vi "test.vi"   [LabVIEW 2019]
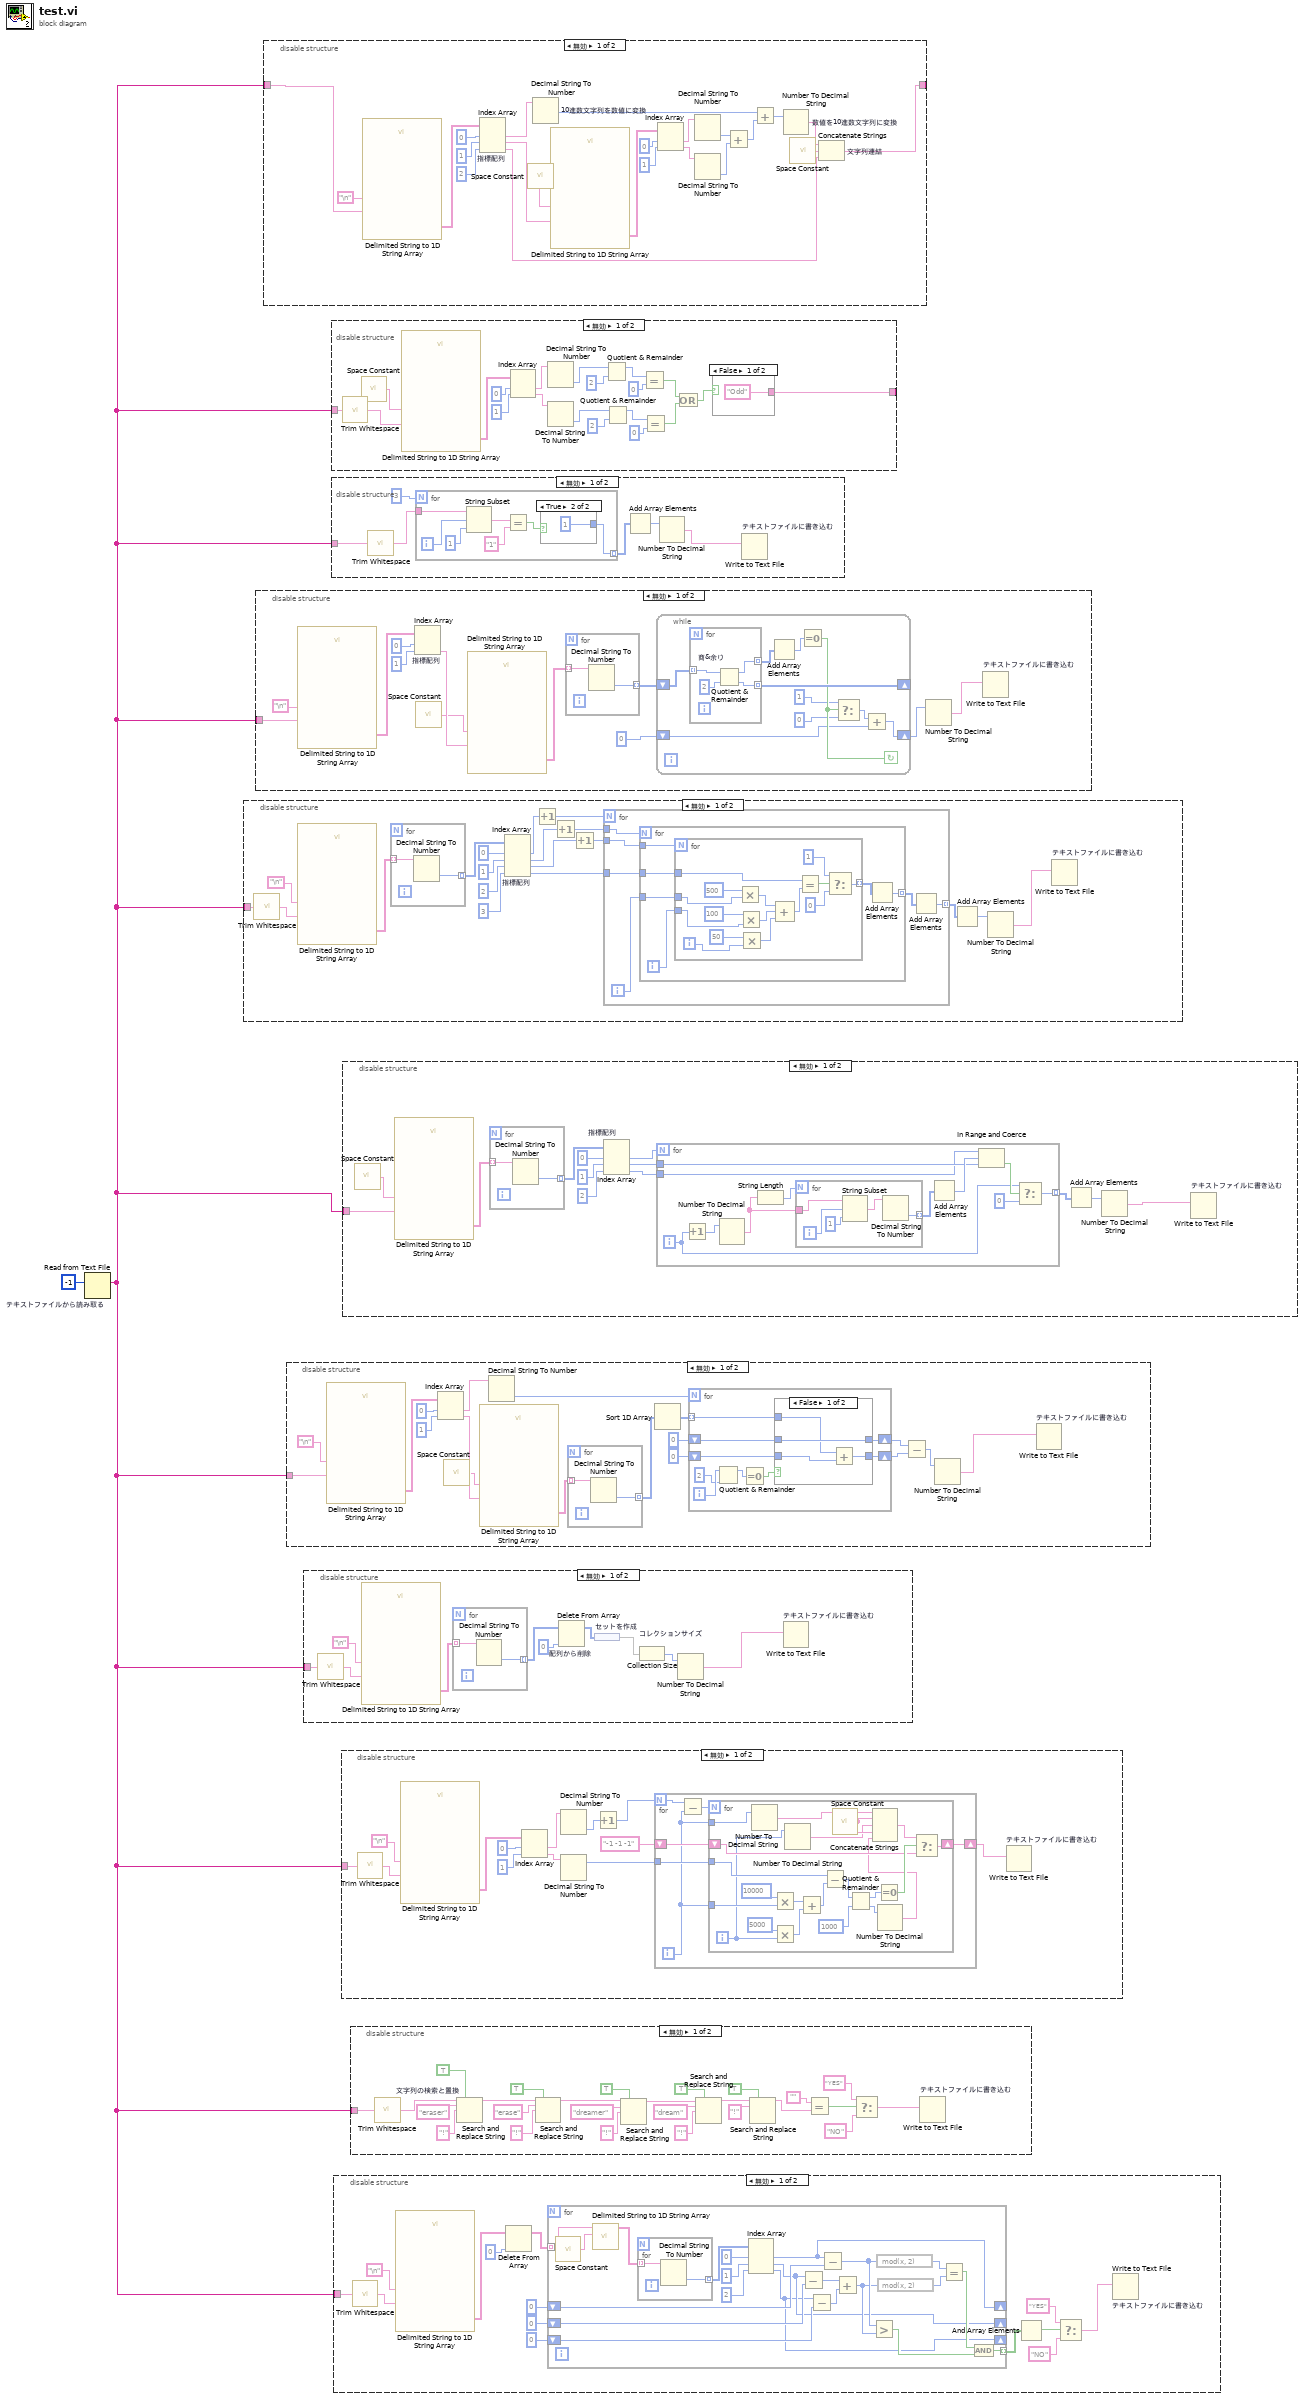
[diagram p0: block diagram]
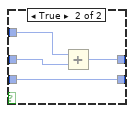
[diagram p7: hidden frame]
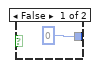
[diagram p11: hidden frame]
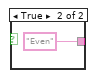
[diagram p13: hidden frame]
diagram:
  n1 = Read from Text File "テキストファイルから読み取る"(count=-1) -> (text=w1:string)  [unwired: 3 in, 3 out]
  n2 = disable-structure shown="無効" {
    disable-tunnel: w1 -> [w21 _]
    frame Disabled {
      n3 = call <vilib>:"Trim Whitespace.vi"("string"=w21) -> ("trimmed string"=w16:string)  [unwired: 1 in]
      n4 = call <vilib>:"Delimited String to 1D String Array.vi"("delimiter"="\n", "delimited string"=w16) -> ("string array"=w13:string[])  [unwired: 9 in]
      n5 = for {
        tunnel: w13 -> [w50] mode=indexing
        tunnel: [w49] -> w12 mode=indexing
        n6 = Decimal String To Number(string=w50) -> (number=w49:i32)  [unwired: 2 in, 1 out]
      }
      n7 = Index Array "指標配列"(array=w12, index #1=0, index #2=1, index #3=2, index #4=3) -> (element #1=w8:i32, element #2=w6:i32, element #3=w4:i32, element #4=w11:i32)
      n8 = Increment(x=w8) -> (x+1=w7:i32)
      n9 = Increment(x=w6) -> (x+1=w5:i32)
      n10 = Increment(x=w4) -> (x+1=w3:i32)
      n11 = for {
        N: w7 -> [_]
        tunnel: w5 -> [w27]
        tunnel: w3 -> [w26]
        tunnel: w11 -> [w25]
        tunnel: [w22] -> w10 mode=indexing
        i -> [w24]
        n12 = for {
          N: w27 -> [_]
          tunnel: w26 -> [w33]
          tunnel: w25 -> [w32]
          tunnel: w24 -> [w31]
          tunnel: [w28] -> w23 mode=indexing
          i -> [w30]
          n13 = for {
            N: w33 -> [_]
            tunnel: w32 -> [w39]
            tunnel: w31 -> [w47]
            tunnel: w30 -> [w45]
            tunnel: [w35] -> w29 mode=indexing
            i -> [w43]
            n14 = Multiply(x=500, y=w47) -> (x*y=w42:i32)
            n15 = Multiply(x=100, y=w45) -> (x*y=w41:i32)
            n16 = Multiply(x=50, y=w43) -> (x*y=w40:i32)
            n17 = Compound Arithmetic op=ADD(w42, w41, w40) -> (w34:i32)
            n18 = Equal?(x=w39, y=w34) -> (x = y?=w38:bool)
            n19 = Select(t=1, s=w38, f=0) -> (s? t:f=w35:i32)
          }
          n20 = Add Array Elements(numeric array=w29) -> (sum=w28:i32)
        }
        n21 = Add Array Elements(numeric array=w23) -> (sum=w22:i32)
      }
      n22 = Add Array Elements(numeric array=w10) -> (sum=w9:i32)
      n23 = Number To Decimal String(number=w9) -> (decimal integer string=w20:string)  [unwired: 1 in]
      n24 = Write to Text File "テキストファイルに書き込む"(text=w20) -> ()  [unwired: 3 in, 3 out]
    }
    frame Enabled {
    }
  }
  n25 = disable-structure shown="無効" {
    disable-tunnel: w1 -> [w62 _]
    frame Disabled {
      n26 = call <vilib>:"Delimited String to 1D String Array.vi"("delimiter"="\n", "delimited string"=w62) -> ("string array"=w57:string[])  [unwired: 9 in]
      n27 = Index Array "指標配列"(array=w57, index #1=0, index #2=1) -> (element #2=w56:string)  [unwired: 1 out]
      n28 = call <vilib>:"Space Constant.vi"() -> ("String"=w55:string)
      n29 = call <vilib>:"Delimited String to 1D String Array.vi"("delimiter"=w55, "delimited string"=w56) -> ("string array"=w54:string[])  [unwired: 9 in]
      n30 = for {
        tunnel: w54 -> [w64] mode=indexing
        tunnel: [w63] -> w53 mode=indexing
        n31 = Decimal String To Number(string=w64) -> (number=w63:i32)  [unwired: 2 in, 1 out]
      }
      n32 = while {
        shift-right: [w72] -> _
        shift-left: w53 -> [w74]
        shift-right: [w65] -> w51
        shift-left: 0 -> [w66]
        stop <- w70 continue-if-true
        n33 = for {
          tunnel: w74 -> [w78] mode=indexing
          tunnel: [w76] -> w72 mode=indexing
          tunnel: [w75] -> w73 mode=indexing
          n34 = Quotient & Remainder "商&余り"(x=w78, y=2) -> (x-y*floor(x/y)=w75:i32, floor(x/y)=w76:i32)
        }
        n35 = Add Array Elements(numeric array=w73) -> (sum=w71:i32)
        n36 = Equal To 0?(x=w71) -> (x = 0?=w70:bool)
        n37 = Select(t=1, s=w70, f=0) -> (s? t:f=w67:i32)
        n38 = Add(x=w67, y=w66) -> (x+y=w65:i32)
      }
      n39 = Number To Decimal String(number=w51) -> (decimal integer string=w61:string)  [unwired: 1 in]
      n40 = Write to Text File "テキストファイルに書き込む"(text=w61) -> ()  [unwired: 3 in, 3 out]
    }
    frame Enabled {
    }
  }
  n41 = disable-structure shown="無効" {
    disable-tunnel: w1 -> [w101 _]
    disable-tunnel: [w79 _] -> _
    frame Disabled {
      n42 = call <vilib>:"Delimited String to 1D String Array.vi"("delimiter"="\n", "delimited string"=w101) -> ("string array"=w100:string[])  [unwired: 9 in]
      n43 = Index Array "指標配列"(array=w100, index #1=0, index #2=1, index #3=2) -> (element #1=w95:string, element #2=w94:string, element #3=w80:string)
      n44 = call <vilib>:"Space Constant.vi"() -> ("String"=w93:string)
      n45 = Decimal String To Number "10進数文字列を数値に変換"(string=w95) -> (number=w86:i32)  [unwired: 2 in, 1 out]
      n46 = call <vilib>:"Delimited String to 1D String Array.vi"("delimiter"=w93, "delimited string"=w94) -> ("string array"=w92:string[])  [unwired: 9 in]
      n47 = Index Array(array=w92, index #1=0, index #2=1) -> (element #1=w89:string, element #2=w88:string)
      n48 = Decimal String To Number(string=w89) -> (number=w85:i32)  [unwired: 2 in, 1 out]
      n49 = Decimal String To Number(string=w88) -> (number=w84:i32)  [unwired: 2 in, 1 out]
      n50 = Add(x=w85, y=w84) -> (x+y=w87:i32)
      n51 = Add(x=w86, y=w87) -> (x+y=w83:i32)
      n52 = Number To Decimal String "数値を10進数文字列に変換"(number=w83) -> (decimal integer string=w82:string)  [unwired: 1 in]
      n53 = call <vilib>:"Space Constant.vi"() -> ("String"=w81:string)
      n54 = Concatenate Strings "文字列連結"(w82, w81, w80) -> (w79:string)
    }
    frame Enabled {
    }
  }
  n55 = disable-structure shown="無効" {
    disable-tunnel: w1 -> [w118 _]
    frame Disabled {
      n56 = call <vilib>:"Delimited String to 1D String Array.vi"("delimiter"="\n", "delimited string"=w118) -> ("string array"=w117:string[])  [unwired: 9 in]
      n57 = Index Array ("指標配列")(array=w117, index #1=0, index #2=1) -> (element #1=w113:string, element #2=w112:string)
      n58 = call <vilib>:"Space Constant.vi"() -> ("String"=w111:string)
      n59 = call <vilib>:"Delimited String to 1D String Array.vi"("delimiter"=w111, "delimited string"=w112) -> ("string array"=w110:string[])  [unwired: 9 in]
      n60 = Decimal String To Number(string=w113) -> (number=w109:i32)  [unwired: 2 in, 1 out]
      n61 = for {
        tunnel: w110 -> [w121] mode=indexing
        tunnel: [w120] -> w108 mode=indexing
        n62 = Decimal String To Number(string=w121) -> (number=w120:i32)  [unwired: 2 in, 1 out]
      }
      n63 = Sort 1D Array(array=w108) -> (sorted array=w107:i32[])
      n64 = for {
        N: w109 -> [_]
        tunnel: w107 -> [w123] mode=indexing
        shift-right: [w126] -> w104
        shift-left: 0 -> [w127]
        shift-right: [w124] -> w103
        shift-left: 0 -> [w125]
        i -> [w130]
        n65 = Quotient & Remainder(x=w130, y=2) -> (x-y*floor(x/y)=w129:i32)  [unwired: 1 out]
        n66 = Equal To 0?(x=w129) -> (x = 0?=w128:bool)
        n67 = case shown="FALSE" w128 {
          tunnel: w127 -> [w134 w138]
          tunnel: [w134 w136] -> w126
          tunnel: w125 -> [w133 w137]
          tunnel: [w132 w137] -> w124
          tunnel: w123 -> [w131 w135]
          frame False {
            n68 = Add(x=w131, y=w133) -> (x+y=w132:i32)
          }
          frame True {
            n69 = Add(x=w135, y=w138) -> (x+y=w136:i32)
          }
        }
      }
      n70 = Subtract(x=w104, y=w103) -> (x-y=w102:i32)
      n71 = Number To Decimal String(number=w102) -> (decimal integer string=w119:string)  [unwired: 1 in]
      n72 = Write to Text File "テキストファイルに書き込む"(text=w119) -> ()  [unwired: 3 in, 3 out]
    }
    frame Enabled {
    }
  }
  n73 = disable-structure shown="無効" {
    disable-tunnel: w1 -> [w147 _]
    frame Disabled {
      n74 = call <vilib>:"Trim Whitespace.vi"("string"=w147) -> ("trimmed string"=w146:string)  [unwired: 1 in]
      n75 = call <vilib>:"Delimited String to 1D String Array.vi"("delimiter"="\n", "delimited string"=w146) -> ("string array"=w143:string[])  [unwired: 9 in]
      n76 = for {
        tunnel: w143 -> [w150] mode=indexing
        tunnel: [w149] -> w142 mode=indexing
        n77 = Decimal String To Number(string=w150) -> (number=w149:i32)  [unwired: 2 in, 1 out]
      }
      n78 = Delete From Array "配列から削除"(array=w142, index=0) -> (array with subset deleted=w141:i32[])  [unwired: 1 in, 1 out]
      n79 = node "セットを作成"(w141) -> (w140:set{i32[]})
      n80 = Collection Size "コレクションサイズ"(1:w140) -> (0:w139:i32)
      n81 = Number To Decimal String(number=w139) -> (decimal integer string=w148:string)  [unwired: 1 in]
      n82 = Write to Text File "テキストファイルに書き込む"(text=w148) -> ()  [unwired: 3 in, 3 out]
    }
    frame Enabled {
    }
  }
  n83 = disable-structure shown="無効" {
    disable-tunnel: w1 -> [w152 _]
    disable-tunnel: [w151 _] -> _
    frame Disabled {
      n84 = call <vilib>:"Trim Whitespace.vi"("string"=w152) -> ("trimmed string"=w169:string)  [unwired: 1 in]
      n85 = call <vilib>:"Space Constant.vi"() -> ("String"=w170:string)
      n86 = call <vilib>:"Delimited String to 1D String Array.vi"("delimiter"=w170, "delimited string"=w169) -> ("string array"=w164:string[])  [unwired: 9 in]
      n87 = Index Array(array=w164, index #1=0, index #2=1) -> (element #1=w167:string, element #2=w168:string)
      n88 = Decimal String To Number(string=w167) -> (number=w163:i32)  [unwired: 2 in, 1 out]
      n89 = Decimal String To Number(string=w168) -> (number=w157:i32)  [unwired: 2 in, 1 out]
      n90 = Quotient & Remainder(x=w163, y=2) -> (x-y*floor(x/y)=w160:i32)  [unwired: 1 out]
      n91 = Quotient & Remainder(x=w157, y=2) -> (x-y*floor(x/y)=w156:i32)  [unwired: 1 out]
      n92 = Equal?(x=w160, y=0) -> (x = y?=w155:bool)
      n93 = Equal?(x=w156, y=0) -> (x = y?=w154:bool)
      n94 = Or(x=w155, y=w154) -> (x .or. y?=w153:bool)
      n95 = case shown="FALSE" w153 {
        tunnel: ["Odd" "Even"] -> w151
        frame False {
        }
        frame True {
        }
      }
    }
    frame Enabled {
    }
  }
  n96 = disable-structure shown="無効" {
    disable-tunnel: w1 -> [w178 _]
    frame Disabled {
      n97 = call <vilib>:"Trim Whitespace.vi"("string"=w178) -> ("trimmed string"=w176:string)  [unwired: 1 in]
      n98 = for {
        N: 3 -> [_]
        tunnel: w176 -> [w183]
        tunnel: [w179] -> w174 mode=indexing
        i -> [w181]
        n99 = String Subset(string=w183, offset (0)=w181, length (rest)=1) -> (substring=w182:string)
        n100 = Equal?(x=w182, y="1") -> (x = y?=w184:bool)
        n101 = case shown="TRUE" w184 {
          tunnel: [0 1] -> w179
          frame False {
          }
          frame True {
          }
        }
      }
      n102 = Add Array Elements(numeric array=w174) -> (sum=w173:i32)
      n103 = Number To Decimal String(number=w173) -> (decimal integer string=w177:string)  [unwired: 1 in]
      n104 = Write to Text File "テキストファイルに書き込む"(text=w177) -> ()  [unwired: 3 in, 3 out]
    }
    frame Enabled {
    }
  }
  n105 = disable-structure shown="無効" {
    disable-tunnel: w1 -> [w201 _]
    frame Disabled {
      n106 = call <vilib>:"Trim Whitespace.vi"("string"=w201) -> ("trimmed string"=w199:string)  [unwired: 1 in]
      n107 = call <vilib>:"Delimited String to 1D String Array.vi"("delimiter"="\n", "delimited string"=w199) -> ("string array"=w196:string[])  [unwired: 9 in]
      n108 = Delete From Array ("配列から削除")(array=w196, index=0) -> (array with subset deleted=w195:string[])  [unwired: 1 in, 1 out]
      n109 = for {
        tunnel: w195 -> [w223] mode=indexing
        shift-right: [w215] -> _
        shift-left: 0 -> [w216]
        shift-right: [w203] -> _
        shift-left: 0 -> [w214]
        shift-right: [w202] -> _
        shift-left: 0 -> [w213]
        tunnel: [w204] -> w191 mode=indexing
        n110 = call <vilib>:"Space Constant.vi"() -> ("String"=w222:string)
        n111 = call <vilib>:"Delimited String to 1D String Array.vi"("delimiter"=w222, "delimited string"=w223) -> ("string array"=w221:string[])  [unwired: 9 in]
        n112 = for {
          tunnel: w221 -> [w225] mode=indexing
          tunnel: [w224] -> w219 mode=indexing
          n113 = Decimal String To Number(string=w225) -> (number=w224:i32)  [unwired: 2 in, 1 out]
        }
        n114 = Index Array ("指標配列")(array=w219, index #1=0, index #2=1, index #3=2) -> (element #1=w215:i32, element #2=w203:i32, element #3=w202:i32)
        n115 = Subtract(x=w203, y=w214) -> (x-y=w212:i32)
        n116 = Subtract(x=w202, y=w213) -> (x-y=w211:i32)
        n117 = Subtract(x=w215, y=w216) -> (x-y=w208:i32)
        n118 = Add(x=w212, y=w211) -> (x+y=w207:i32)
        n119 = Greater?(x=w208, y=w207) -> (0:w205:bool)
        n120 = expression code="mod(x, 2)"(w208) -> (w210:i32)
        n121 = expression code="mod(x, 2)"(w207) -> (w209:i32)
        n122 = Equal?(x=w210, y=w209) -> (x = y?=w206:bool)
        n123 = And(x=w206, y=w205) -> (x .and. y?=w204:bool)
      }
      n124 = And Array Elements(Boolean array=w191) -> (logical AND=w188:bool)
      n125 = Select(t="YES" ("検索文字列"), s=w188, f="NO" ("検索文字列")) -> (s? t:f=w200:string)
      n126 = Write to Text File "テキストファイルに書き込む"(text=w200) -> ()  [unwired: 3 in, 3 out]
    }
    frame Enabled {
    }
  }
  n127 = disable-structure shown="無効" {
    disable-tunnel: w1 -> [w237 _]
    frame Disabled {
      n128 = call <vilib>:"Trim Whitespace.vi"("string"=w237) -> ("trimmed string"=w235:string)  [unwired: 1 in]
      n129 = call <vilib>:"Delimited String to 1D String Array.vi"("delimiter"="\n", "delimited string"=w235) -> ("string array"=w232:string[])  [unwired: 9 in]
      n130 = Index Array ("指標配列")(array=w232, index #1=0, index #2=1) -> (element #1=w231:string, element #2=w230:string)
      n131 = Decimal String To Number(string=w231) -> (number=w228:i32)  [unwired: 2 in, 1 out]
      n132 = Decimal String To Number(string=w230) -> (offset past number=w227:i32)  [unwired: 2 in, 1 out]
      n133 = Increment(x=w228) -> (x+1=w229:i32)
      n134 = for {
        N: w229 -> [w244]
        tunnel: w227 -> [w242]
        shift-right: [w239] -> w238
        shift-left: "-1 -1 -1" -> [w241]
        i -> [w240]
        n135 = Subtract(x=w244, y=w240) -> (x-y=w243:i32)
        n136 = for {
          N: w243 -> [_]
          tunnel: w242 -> [w260]
          tunnel: w240 -> [w264]
          shift-right: [w254] -> w239
          shift-left: w241 -> [w253]
          tunnel: w240 -> [w252]
          i -> [w248]
          n137 = Number To Decimal String(number=w252) -> (decimal integer string=w251:string)  [unwired: 1 in]
          n138 = Multiply(x=10000, y=w264) -> (x*y=w262:i32)
          n139 = Multiply(x=5000, y=w248) -> (x*y=w261:i32)
          n140 = Number To Decimal String(number=w248) -> (decimal integer string=w247:string)  [unwired: 1 in]
          n141 = Add(x=w262, y=w261) -> (x+y=w259:i32)
          n142 = Subtract(x=w260, y=w259) -> (x-y=w258:i32)
          n143 = call <vilib>:"Space Constant.vi"() -> ("String"=w250:string)
          n144 = Quotient & Remainder(x=w258, y=1000) -> (x-y*floor(x/y)=w256:i32, floor(x/y)=w246:i32)
          n145 = Equal To 0?(x=w256) -> (x = 0?=w255:bool)
          n146 = Number To Decimal String(number=w246) -> (decimal integer string=w245:string)  [unwired: 1 in]
          n147 = Concatenate Strings(w251, w250, w247, w250, w245) -> (w249:string)
          n148 = Select(t=w249, s=w255, f=w253) -> (s? t:f=w254:string)
        }
      }
      n149 = Write to Text File "テキストファイルに書き込む"(text=w238) -> ()  [unwired: 3 in, 3 out]
    }
    frame Enabled {
    }
  }
  n150 = disable-structure shown="無効" {
    disable-tunnel: w1 -> [w278 _]
    frame Disabled {
      n151 = call <vilib>:"Space Constant.vi"() -> ("String"=w276:string)
      n152 = call <vilib>:"Delimited String to 1D String Array.vi"("delimiter"=w276, "delimited string"=w278) -> ("string array"=w275:string[])  [unwired: 9 in]
      n153 = for {
        tunnel: w275 -> [w296] mode=indexing
        tunnel: [w295] -> w272 mode=indexing
        n154 = Decimal String To Number(string=w296) -> (number=w295:i32)  [unwired: 2 in, 1 out]
      }
      n155 = Index Array "指標配列"(array=w272, index #1=0, index #2=1, index #3=2) -> (element #1=w270:i32, element #2=w269:i32, element #3=w268:i32)
      n156 = for {
        N: w270 -> [_]
        tunnel: w269 -> [w284]
        tunnel: w268 -> [w283]
        tunnel: [w279] -> w267 mode=indexing
        i -> [w281]
        n157 = Increment(x=w281) -> (x+1=w289:i32)
        n158 = Number To Decimal String(number=w289) -> (decimal integer string=w287:string)  [unwired: 1 in]
        n159 = String Length(string=w287) -> (length=w288:i32)
        n160 = for {
          N: w288 -> [_]
          tunnel: w287 -> [w294]
          tunnel: [w290] -> w286 mode=indexing
          i -> [w292]
          n161 = String Subset(string=w294, offset (0)=w292, length (rest)=1 ("長さ (残り)")) -> (substring=w291:string)
          n162 = Decimal String To Number(string=w291) -> (number=w290:i32)  [unwired: 2 in, 1 out]
        }
        n163 = Add Array Elements(numeric array=w286) -> (sum=w285:i32)
        n164 = In Range and Coerce(upper limit=w283, x=w285, lower limit=w284) -> (In Range?=w282:bool)  [unwired: 1 out]
        n165 = Select(t=w281, s=w282, f=0) -> (s? t:f=w279:i32)
      }
      n166 = Add Array Elements(numeric array=w267) -> (sum=w266:i32)
      n167 = Number To Decimal String(number=w266) -> (decimal integer string=w277:string)  [unwired: 1 in]
      n168 = Write to Text File "テキストファイルに書き込む"(text=w277) -> ()  [unwired: 3 in, 3 out]
    }
    frame Enabled {
    }
  }
  n169 = disable-structure shown="無効" {
    disable-tunnel: w1 -> [w321 _]
    frame Disabled {
      n170 = call <vilib>:"Trim Whitespace.vi"("string"=w321) -> ("trimmed string"=w317:string)  [unwired: 1 in]
      n171 = Search and Replace String "文字列の検索と置換"(replace all?=TRUE ("すべて置換? (F)"), input string=w317, search string="eraser" ("検索文字列"), replace string="!" ("置換文字列 (\"\")")) -> (result string=w307:string)  [unwired: 4 in, 3 out]
      n172 = Search and Replace String ("文字列の検索と置換")(replace all?=TRUE ("すべて置換? (F)"), input string=w307, search string="erase" ("検索文字列"), replace string="!" ("置換文字列 (\"\")")) -> (result string=w306:string)  [unwired: 4 in, 3 out]
      n173 = Search and Replace String ("文字列の検索と置換")(replace all?=TRUE ("すべて置換? (F)"), input string=w306, search string="dreamer" ("検索文字列"), replace string="!" ("置換文字列 (\"\")")) -> (result string=w305:string)  [unwired: 4 in, 3 out]
      n174 = Search and Replace String ("文字列の検索と置換")(replace all?=TRUE ("すべて置換? (F)"), input string=w305, search string="dream" ("検索文字列"), replace string="!" ("置換文字列 (\"\")")) -> (result string=w302:string)  [unwired: 4 in, 3 out]
      n175 = Search and Replace String ("文字列の検索と置換")(replace all?=TRUE ("すべて置換? (F)"), input string=w302, search string="!" ("検索文字列")) -> (result string=w300:string)  [unwired: 5 in, 3 out]
      n176 = Equal?(x="", y=w300) -> (x = y?=w299:bool)
      n177 = Select(t="YES" ("検索文字列"), s=w299, f="NO" ("検索文字列")) -> (s? t:f=w322:string)
      n178 = Write to Text File "テキストファイルに書き込む"(text=w322) -> ()  [unwired: 3 in, 3 out]
    }
    frame Enabled {
    }
  }
